vi "Draw Flat Top Filled Triangle 1D.vi"(4 "Fill Colour":u32(colorbox), 6 "Enable Alpha Blending (F)":bool, 7 "Alpha":dbl, 8 "Vertex 3":T1={"Position"={"x"=0.0, "y"=0.0, "z"=0.0}, "UV"={"u"=0.0, "v"=0.0}, "Colour"=12517256} {"UV"."v" min=0 max=1 step=0.1; "UV"."u" min=0 max=1 step=0.1}, 9 "Vertex 2":T1={"Position"={"x"=0.0, "y"=0.0, "z"=0.0}, "UV"={"u"=0.0, "v"=0.0}, "Colour"=12517256} {"UV"."v" min=0 max=1 step=0.1; "UV"."u" min=0 max=1 step=0.1}, 10 "Vertex 1":T1={"Position"={"x"=0.0, "y"=0.0, "z"=0.0}, "UV"={"u"=0.0, "v"=0.0}, "Colour"=12517256} {"UV"."v" min=0 max=1 step=0.1; "UV"."u" min=0 max=1 step=0.1}, 11 "Pixel Data in":u32[](array[numeric])) -> (3 "Pixel Data out":u32[](array[numeric]))   [LabVIEW 2020, in "Raster (FPGA).lvlib"]
uses:
  Raster (FPGA).lvlib
  Point 2D (I32).ctl
  Method.ctl
  3D/Vector 3D.ctl
  3D/3D (FPGA).lvlib
  UV.ctl
  3D/Vertex.ctl
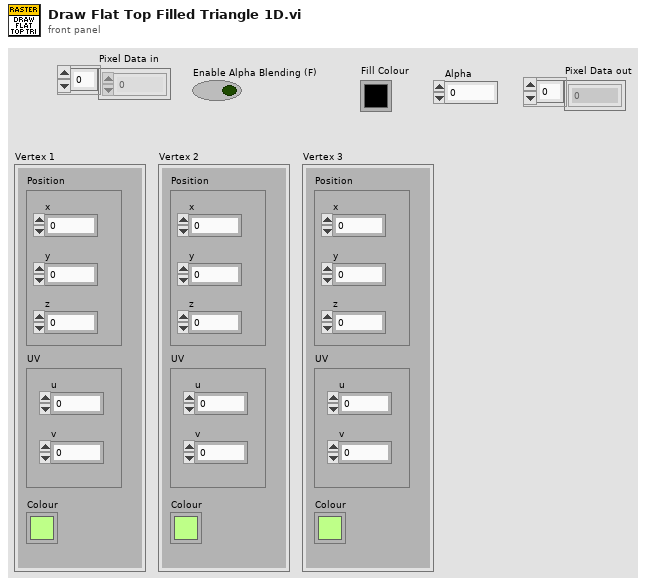
[diagram p1: front panel]
types:
  T1 = typedef "3D (FPGA).lvlib/Vertex.ctl" = cluster{"Position":T2, "UV":T3, "Colour":u32}
  T2 = typedef "3D (FPGA).lvlib/Vector 3D.ctl" = cluster{"x":sgl, "y":sgl, "z":sgl}
  T3 = typedef "Raster (FPGA).lvlib/UV.ctl" = cluster{"u":sgl, "v":sgl}
  T4 = typedef "Raster (FPGA).lvlib/Point 2D (I32).ctl" = cluster{"x":i32, "y":i32}
  T5 = typedef "Raster (FPGA).lvlib/Method.ctl" = enum16{"Per item", "Row", "Replace Array Subset", "MoveBlock", " MoveBlock2 "}
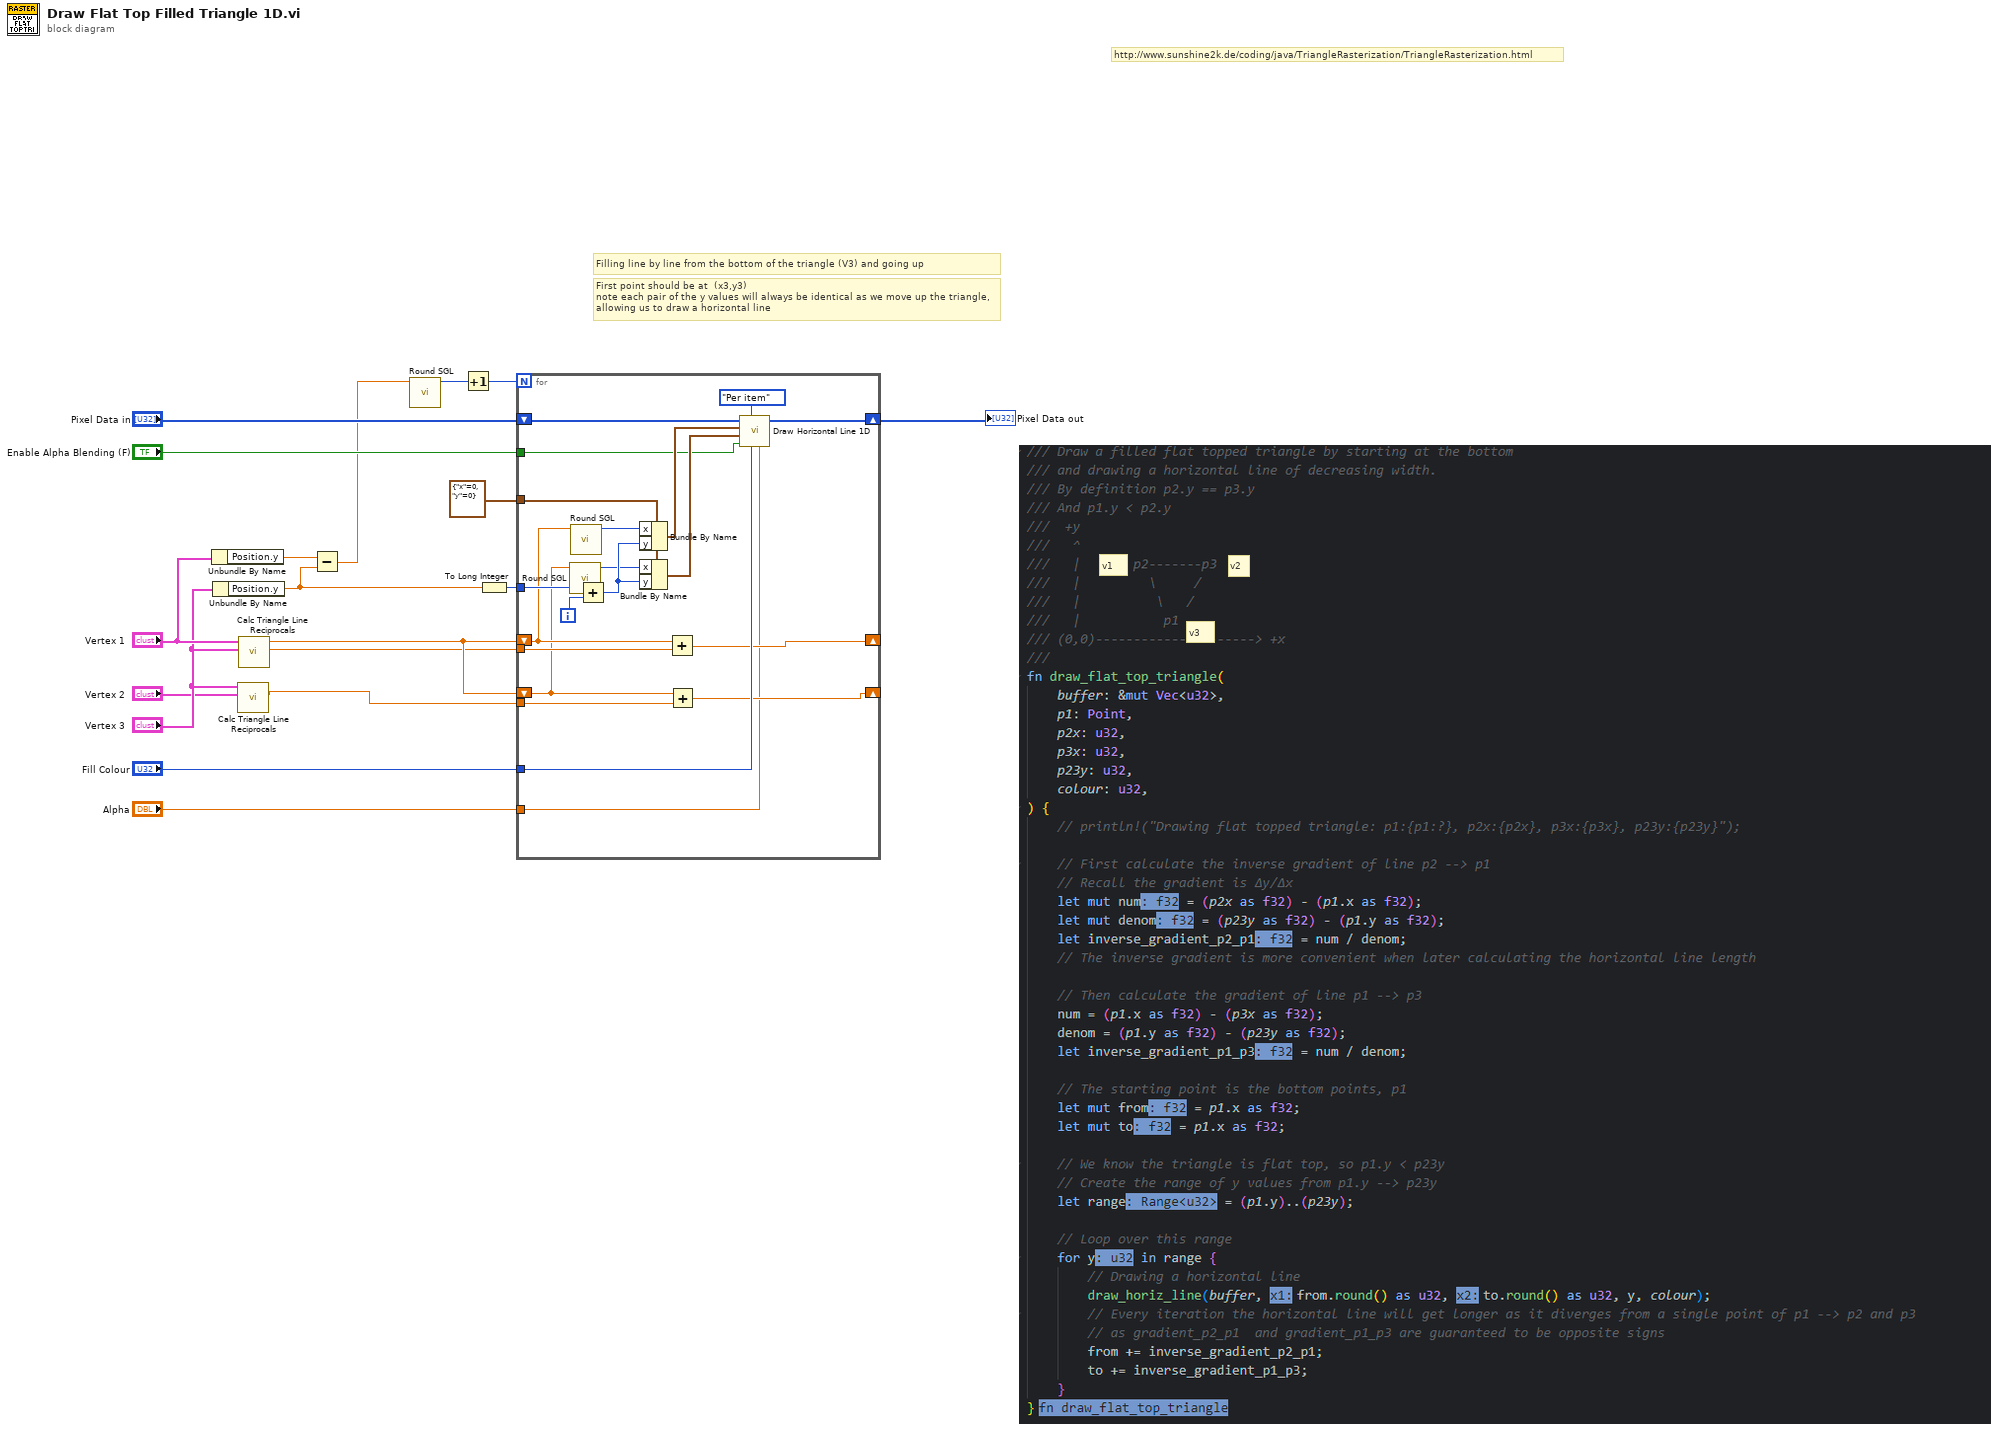
[diagram p0: block diagram]
diagram:
  # "v3"
  # "v2"
  # "v1"
  # "First point should be at  (x3,y3) \nnote each pair of the y values will always be identical as we move up the triangle, allowing us to draw a horizontal line"
  # "Filling line by line from the bottom of the triangle (V3) and going up"
  # "http://www.sunshine2k.de/coding/java/TriangleRasterization/TriangleRasterization.html"
  n1 = Unbundle By Name("Vertex 1") -> ("Position.y"=w10:sgl)
  n2 = Unbundle By Name("Vertex 3") -> ("Position.y"=w9:sgl)
  n3 = call "Calc Triangle Line Reciprocals.vi"("Vertex 2"="Vertex 2", "Vertex 1"="Vertex 3") -> ("Delta x"=w3:sgl)  [unwired: 8 in, 1 out]
  n4 = call "Calc Triangle Line Reciprocals.vi"("Vertex 2"="Vertex 3", "Vertex 1"="Vertex 1") -> ("Delta x"=w4:sgl, "Starting x"=w5:sgl)  [unwired: 8 in]
  n5 = Subtract(x=w10, y=w9) -> (x-y=w2:sgl)
  n6 = call "Round SGL.vi"("SGL"=w2) -> ("I32"=w1:i32)  [unwired: 10 in]
  n7 = Increment(x=w1) -> (x+1=w12:i32)
  n8 = To Long Integer(number=w9) -> (32bit integer=w16:i32)
  n9 = for {
    N: w12 -> [_]
    tunnel: T4 {"x"=0, "y"=0} ("Point 1") -> [w38]
    tunnel: "Fill Colour" -> [w35]
    shift-right: [w30] -> _
    shift-left: w5 -> [w22]
    shift-right: [w31] -> _
    shift-left: w5 -> [w20]
    tunnel: w16 -> [w33]
    tunnel: w4 -> [w32]
    tunnel: w3 -> [w29]
    shift-right: [w26] -> w11
    shift-left: "Pixel Data in" -> [w27]
    tunnel: "Enable Alpha Blending (F)" -> [w24]
    tunnel: "Alpha" -> [w23]
    i -> [w28]
    n10 = call "Round SGL.vi"("SGL"=w20) -> ("I32"=w19:i32)  [unwired: 10 in]
    n11 = call "Round SGL.vi"("SGL"=w22) -> ("I32"=w21:i32)  [unwired: 10 in]
    n12 = Add(x=w33, y=w28) -> (x+y=w34:i32)
    n13 = Bundle By Name(cluster=w38, "x"=w21, "y"=w34) -> (w37:T4)
    n14 = Bundle By Name(cluster=w38, "x"=w19, "y"=w34) -> (w36:T4)
    n15 = Add(x=w22, y=w32) -> (x+y=w30:sgl)
    n16 = Add(x=w20, y=w29) -> (x+y=w31:sgl)
    n17 = call "Draw Horizontal Line 1D.vi"("Alpha"=w23, "Colour"=w35, "Method"=Method."Per item", "Enable Alpha Blending (F)"=w24, "Point 2"=w36, "Point 1"=w37, "Pixel Data in"=w27) -> ("Pixel Data out"=w26:u32[])  [unwired: 4 in]
  }
  "Pixel Data out" <- w11
